vi "Initialize.vi"(8 "error in (no error)":errorcluster, 11 "Projects in":refnum<class "Projects.lvclass">) -> (0 "error out":errorcluster, 3 "Projects out":refnum<class "Projects.lvclass">)   [LabVIEW 2020, in "Projects.lvclass"]
doc: "Perform any initialization actions necessary for the specific implementations of the class.\nThis implementation clears the Map by writing an empty Map to the project data.\n\n03/2025 Erich Schlieper"
uses:
  Projects.lvclass
  Controls/Project Info.ctl
  Projects.lvclass/Projects.ctl
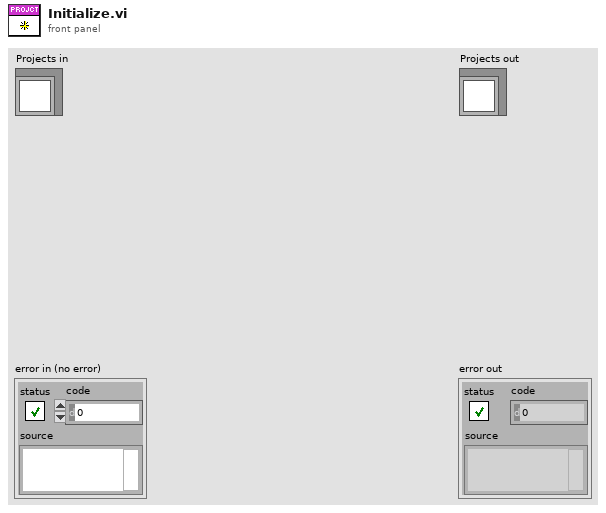
[diagram p1: front panel]
types:
  T1 = typedef "Project Info.ctl" = cluster{"Project Active?":bool, "Tasks":set{string}, "Task Active":map{string, bool}}
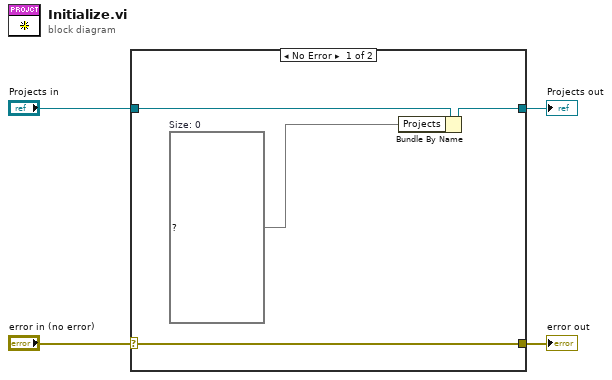
[diagram p0: block diagram]
diagram:
  n1 = case shown="No Error" "error in (no error)" {
    selector: "error in (no error)" -> [w7 w10]
    tunnel: [w7 w10] -> w3
    tunnel: [w6 w9] -> w1
    tunnel: "Projects in" -> [w8 w9]
    frame No Error {
      w5 = map{string, T1} {}  # Size: 0
      n2 = Bundle By Name(cluster=w8, "Projects"=w5) -> (w6:refnum<class "Projects.lvclass">)
    }
    frame Error {
    }
  }
  "error out" <- w3
  "Projects out" <- w1
